vi "ke37xx Reset DMM.vi"(0 "VISA Resource Name":refnum<visa-resource-name>, 7 "Reset All (False)":bool, 11 "error in (no error)":errorcluster) -> (4 "VISA Resource Name Out":refnum<visa-resource-name>, 15 "error out":errorcluster)   [LabVIEW 2009, in "Keithley 3700 Series.lvlib"]
doc: "This VI allows you to reset the DMM aspects of the system for either the currently selected measurement function or for all DMM aspects."
uses:
  <instrlib>/Keithley 3706/Keithley 3700 Series.lvlib
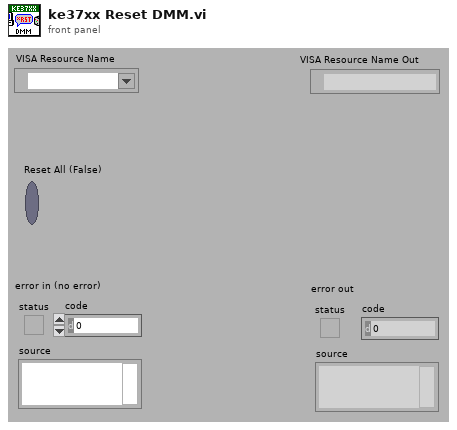
[diagram p1: front panel]
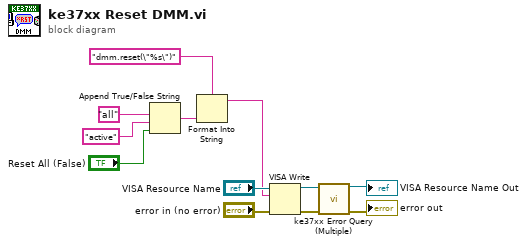
[diagram p0: block diagram]
diagram:
  n1 = Append True/False String(1:"Reset All (False)", 2:"active" ("true string"), 3:"all" ("true string")) -> (0:w4:string)  [unwired: 1 out]
  n2 = Format Into String(format string="dmm.reset(\"%s\")", w4) -> (resulting string=w10:string)  [unwired: 2 in, 1 out]
  n3 = VISA Write(VISA resource name="VISA Resource Name", write buffer=w10, error in (no error)="error in (no error)") -> (VISA resource name out=w9:refnum<visa-resource-name>, error out=w7:errorcluster)  [unwired: 1 out]
  n4 = call <instrlib>:"ke37xx Error Query (Multiple).vi"("VISA resource name"=w9, "error in (no error)"=w7) -> ("VISA resource name out"=→"VISA Resource Name Out":refnum<visa-resource-name>, "error out"=→"error out":errorcluster)  [unwired: 12 out]
